vi "Offset from point Given Distance.vi"(9 "Bearing (clockwise from North)":dbl, 10 "Distance (km)":dbl, 11 "Origin Point":T1 {"Latitude" format="%#_10g"; "Longitude" format="%#_10g"}) -> (0 "Lat of new point":dbl, 1 "Lon of new point":dbl, 2 "Lat Offset":dbl, 3 "Lon Offset":dbl)   [LabVIEW 2014]
uses:
  Controls/PointLatLon.ctl
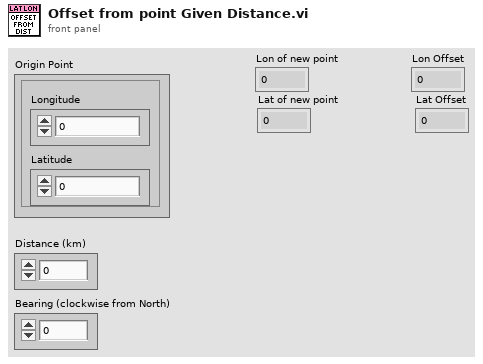
[diagram p1: front panel]
types:
  T1 = typedef "PointLatLon.ctl" = cluster{"Longitude":dbl, "Latitude":dbl}
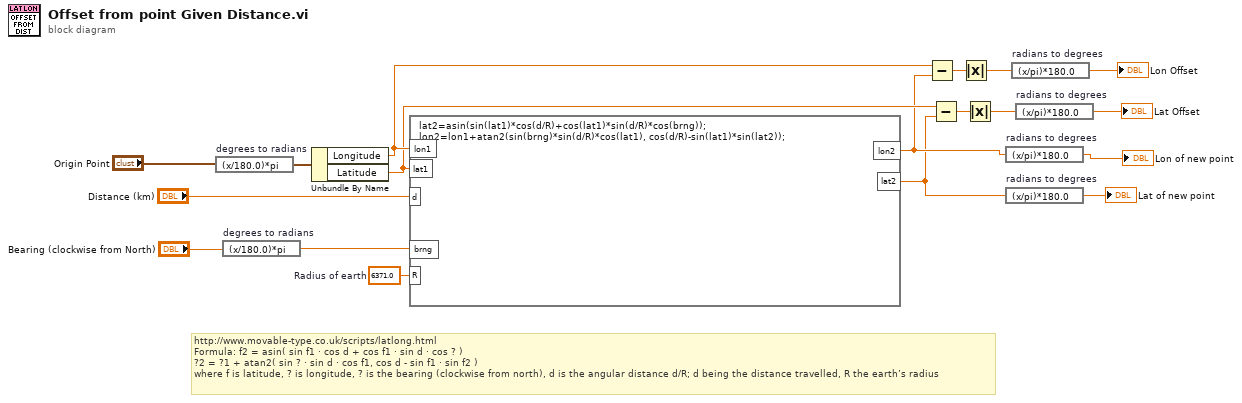
[diagram p0: block diagram]
diagram:
  w14 = 6371.0  # Radius of earth
  # "http://www.movable-type.co.uk/scripts/latlong.html\nFormula:\tf2 = asin( sin f1 · cos d + cos f1 · sin d · cos ? )\n?2 = ?1 + atan2( sin ? · sin d · cos f1, cos d - sin f1 · sin f2 )\nwhere\tf is latitude, ? is longitude, ? is the bearing (clockwise from north), d is the angular distance d/R; d being the distance travelled, R the earth’s radius"
  n1 = expression code="(x/180.0)*pi" "degrees to radians"("Origin Point") -> (w17:T1)
  n2 = expression code="(x/180.0)*pi" "degrees to radians"("Bearing (clockwise from North)") -> (w15:dbl)
  n3 = Unbundle By Name(w17) -> ("Longitude"=w12:dbl, "Latitude"=w5:dbl)
  n4 = formula code="lat2=asin(sin(lat1)*cos(d/R)+cos(lat1)*sin(d/R)*cos(brng));\nlon2=lon1+atan2(sin(brng)*sin(d/R)*cos(lat1), cos(d/R)-sin(lat1)*sin(lat2));"("lon1"=w12, "lat1"=w5, "brng"=w15, "d"="Distance (km)", "R"=w14) -> ("lat2"=w2:dbl, "lon2"=w4:dbl)
  n5 = Subtract(x=w12, y=w4) -> (x-y=w11:dbl)
  n6 = Subtract(x=w5, y=w2) -> (x-y=w6:dbl)
  n7 = Absolute Value(x=w11) -> (abs(x)=w10:dbl)
  n8 = Absolute Value(x=w6) -> (abs(x)=w7:dbl)
  n9 = expression code="(x/pi)*180.0" "radians to degrees"(w4) -> (→"Lon of new point":dbl)
  n10 = expression code="(x/pi)*180.0" "radians to degrees"(w2) -> (→"Lat of new point":dbl)
  n11 = expression code="(x/pi)*180.0" "radians to degrees"(w10) -> (→"Lon Offset":dbl)
  n12 = expression code="(x/pi)*180.0" "radians to degrees"(w7) -> (→"Lat Offset":dbl)
